vi "Flip Lock.vi"(11 "Input":bool) -> (3 "Output":bool)   [LabVIEW 2018]
panel:
  in  "Locked Value":bool
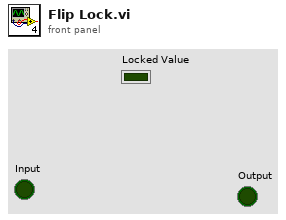
[diagram p1: front panel]
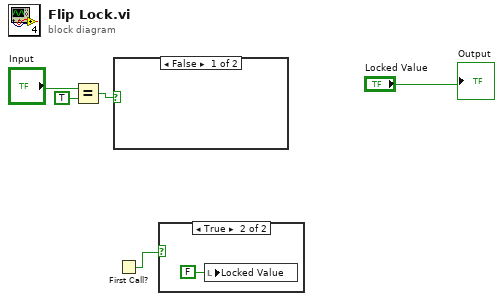
[diagram p0: block diagram]
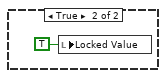
[diagram p3: hidden frame]
diagram:
  n1 = Equal?(x="Input", y=TRUE) -> (x = y?=w3:bool)
  n2 = case shown="False" w3 {
    frame False {
    }
    frame True {
      n3 = local write "Locked Value"(TRUE ("Locked Value")) -> ()
    }
  }
  n4 = First Call?() -> (First Call?: T/F=w1:bool)
  n5 = case shown="True" w1 {
    frame False {
    }
    frame True {
      n6 = local write "Locked Value"(FALSE ("Locked Value")) -> ()
    }
  }
  "Output" <- "Locked Value"
